vi "Send Batch Messages To Specific Target.vi"(6 "Paras In":variant, 7 "Priority":i32, 8 "error in (no error)":errorcluster, 9 "Mail Strategy In":refnum<class "Mail Strategy.lvclass">, 10 "Messages In":refnum<class "Message.lvclass">[](array[class]), 11 "Simple Map Queue Group Messenger in":refnum<class "Simple Map Queue Group Messenger.lvclass">) -> (0 "error out":errorcluster, 3 "Simple Map Queue Group Messenger out":refnum<class "Simple Map Queue Group Messenger.lvclass">)   [LabVIEW 2024, in "Simple Map Queue Group Messenger.lvclass"]
uses:
  Simple Map Queue Group Messenger.lvclass
  Ancestor Class/Message/Message.lvclass
  Ancestor Class/Messenger/Mail Strategy/Mail Strategy.lvclass
  Simple Map Queue Group Messenger.lvclass/Simple Map Queue Group Messenger.ctl
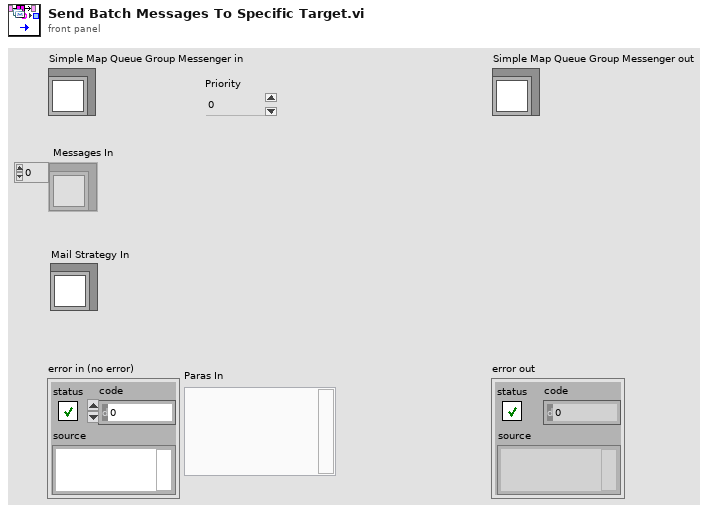
[diagram p1: front panel]
types:
  T1 = typedef "Queue Group Map.ctl" = map{i64, T2[]}
  T2 = typedef "Message Queue.ctl" = refnum<queue>
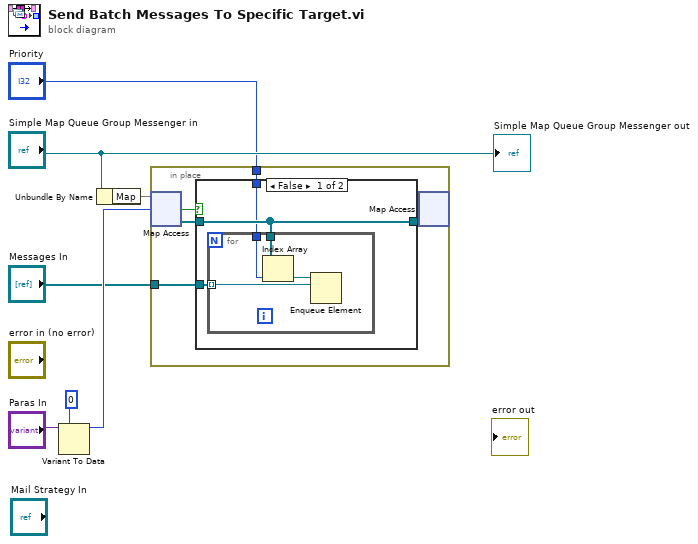
[diagram p0: block diagram]
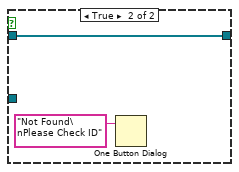
[diagram p2: hidden frame]
diagram:
  n1 = Variant To Data(type=i64 0, Variant="Paras In") -> (data=w5:i64)  [unwired: 1 in, 1 out]
  n2 = Unbundle By Name("Simple Map Queue Group Messenger in") -> ("Map"=w7:T1)
  n3 = in-place {
    in-place-border: "Messages In" -> [w9]
    in-place-border: "Priority" -> [w8]
    n4 = in-place-map #1(w7, w5) -> (w11:T2[], w12:bool)  [unwired: 1 in]
    n5 = case shown="False" w12 {
      tunnel: w11 -> [w15 w20]
      tunnel: [w15 w20] -> w10
      tunnel: w9 -> [w14 _]
      tunnel: w8 -> [w13 _]
      frame False {
        n6 = for {
          tunnel: w15 -> [w18]
          tunnel: w14 -> [w17] mode=indexing
          tunnel: w13 -> [w16]
          n7 = Index Array(array=w18, index=w16) -> (element=w19:T2)
          n8 = Enqueue Element(queue=w19, element=w17) -> ()  [unwired: 2 in, 3 out]
        }
      }
      frame True {
        n9 = One Button Dialog(message="Not Found\nPlease Check ID") -> ()  [unwired: 1 in, 1 out]
      }
    }
    n10 = in-place-map #1(w10) -> ()  [unwired: 1 in, 3 out]
  }
  "Simple Map Queue Group Messenger out" <- "Simple Map Queue Group Messenger in"
